vi "EXDIR-YAML_CheckStringEmptySpaces.vi"(11 "String":string) -> (3 "empty or all spaces":bool)   [LabVIEW 2016]
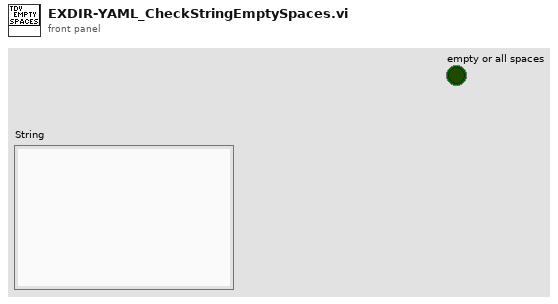
[diagram p1: front panel]
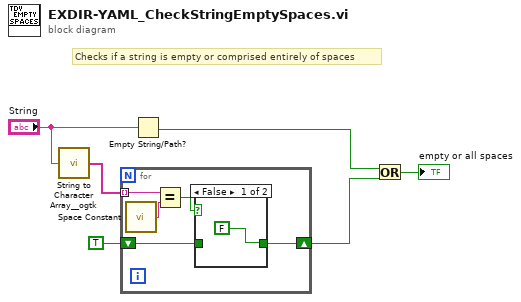
[diagram p0: block diagram]
diagram:
  # "Checks if a string is empty or comprised entirely of spaces"
  n1 = call <userlib>:"String to Character Array__ogtk.vi"("Input String"="String") -> ("Character Array"=w4:string[])
  n2 = for {
    shift-right: [w7] -> w3
    shift-left: TRUE -> [w8]
    tunnel: w4 -> [w10] mode=indexing
    n3 = call <vilib>:"Space Constant.vi"() -> ("String"=w11:string)
    n4 = Equal?(x=w10, y=w11) -> (x = y?=w9:bool)
    n5 = case shown="False" w9 {
      tunnel: w8 -> [_ w13]
      tunnel: [FALSE w13] -> w7
      frame False {
      }
      frame True {
      }
    }
  }
  n6 = Empty String/Path?(string/path="String") -> (empty?=w2:bool)
  n7 = Or(x=w2, y=w3) -> (x .or. y?=→"empty or all spaces":bool)
